vi "Cluster_1.vi"() -> ()   [LabVIEW 2023]
panel:
  out "성적이 업로드 된 클러스터":cluster{"이름":string, "학번":string, "영어점수":dbl}
  out "향상된 영어점수":dbl
  out "영어점수 2":dbl
  out "학번 2":string
  out "이름 2":string
  out "출력 클러스터":cluster{"이름":string, "학번":string, "영어점수":dbl}
  in  "영어점수":dbl
  in  "학번":string
  in  "이름":string
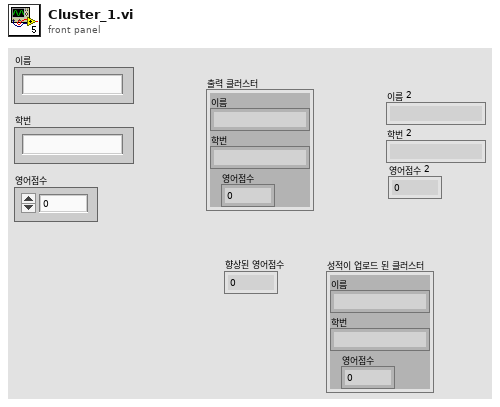
[diagram p1: front panel]
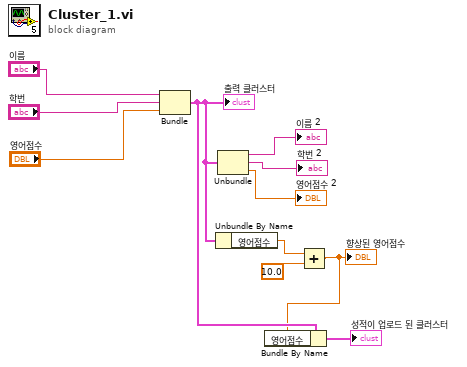
[diagram p0: block diagram]
diagram:
  n1 = Bundle "Bundle"("이름"="이름", "학번"="학번", "영어점수"="영어점수") -> (w3:cluster{"이름":string, "학번":string, "영어점수":dbl})  [unwired: 1 in]
  "출력 클러스터" <- w3
  n2 = Unbundle By Name "Unbundle By Name"(w3) -> ("영어점수"=w5:dbl)
  n3 = Unbundle(w3) -> ("이름"=→"이름 2":string, "학번"=→"학번 2":string, "영어점수"=→"영어점수 2":dbl)
  n4 = Add(x=w5, y=10.0) -> (x+y=w2:dbl)
  "향상된 영어점수" <- w2
  n5 = Bundle By Name "Bundle By Name"(cluster=w3, "영어점수"=w2) -> (→"성적이 업로드 된 클러스터":cluster{"이름":string, "학번":string, "영어점수":dbl})
